vi "Unbox Path.vi"(8 "error in (no error)":errorcluster, 9 "Message":refnum<class "Message.lvclass">) -> (0 "error out":errorcluster, 2 "Message Data":path)   [LabVIEW 2018, in "LapDog.Messaging.v3.NativeTypes.lvlib" / "PathMsg.lvclass"]
doc: "This method is syntactic sugar replacing the often repeated boilerplate code of downcasting a message object to the specific message type and then getting the data from the message.\n\nThe method runs regardless of the error in state."
uses:
  PathMsg.lvclass
  LapDog.Messaging/Message/Message.lvclass
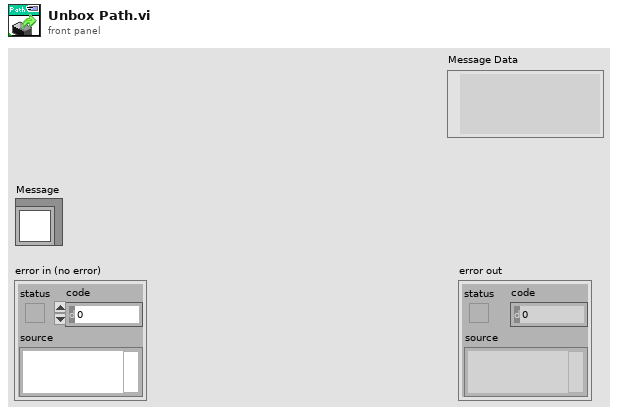
[diagram p1: front panel]
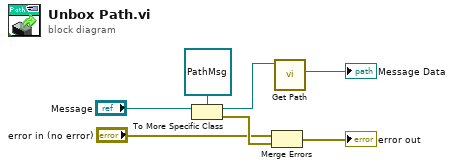
[diagram p0: block diagram]
diagram:
  n1 = To More Specific Class(target class=refnum<class "PathMsg.lvclass"> refnum ("LapDog.Messaging.v3.NativeTypes.lvlib:PathMsg.lvclass"), reference="Message") -> (specific class reference=w2:refnum<class "PathMsg.lvclass">, error out=w7:errorcluster)  [unwired: 1 in]
  n2 = Merge Errors("error in (no error)", w7) -> (→"error out":errorcluster)
  n3 = call-dynamic "Get Path.vi"("PathMsg in"=w2) -> ("Message Data"=→"Message Data":path)  [unwired: 8 in, 2 out]
